vi "Check If Calibration Data Exist.vi"(9 "Set Pressures List":dbl[][](array[numeric])=[[665.1538332158755, 622.4106177021335]], 10 "Mix Cluster":T2, 11 "Calibration Refs":T1) -> (1 "Calibration Data Exists?":bool, 2 "Pressure For Mix 2":dbl[](array[numeric]), 3 "Pressure For Mix 1":dbl[](array[numeric]))   [LabVIEW 2016]
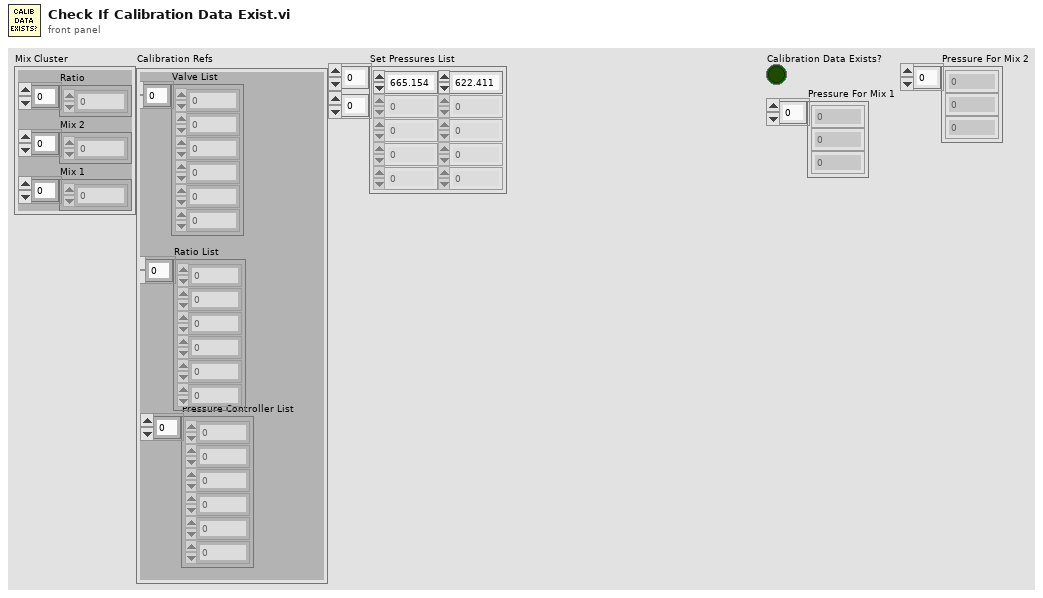
[diagram p1: front panel]
types:
  T1 = cluster{"Pressure Controller List":u8[], "Ratio List":dbl[], "Valve List":u16[]}
  T2 = cluster{"Ratio":dbl[], "Mix 2":u16[], "Mix 1":u16[]}
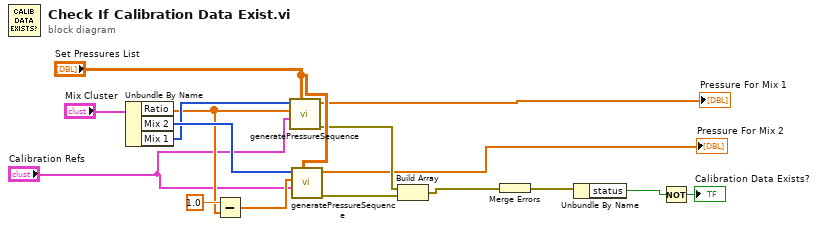
[diagram p0: block diagram]
diagram:
  n1 = Unbundle By Name("Mix Cluster") -> ("Ratio"=w12:dbl[], "Mix 2"=w15:u16[], "Mix 1"=w14:u16[])
  n2 = Subtract(x=1.0, y=w12) -> (x-y=w11:dbl[])
  n3 = call "generatePressureSequence.vi"("Set Pressures List"="Set Pressures List", "Calibration Refs"="Calibration Refs", "Ratio"=w12, "Mix"=w14) -> ("error out"=w7:errorcluster, "Pressure For Mix"=→"Pressure For Mix 1":dbl[])  [unwired: 3 in, 3 out]
  n4 = call "generatePressureSequence.vi"("Set Pressures List"="Set Pressures List", "Calibration Refs"="Calibration Refs", "Ratio"=w11, "Mix"=w15) -> ("error out"=w8:errorcluster, "Pressure For Mix"=→"Pressure For Mix 2":dbl[])  [unwired: 3 in, 3 out]
  n5 = Build Array(w7, w8) -> (w6:errorcluster[])
  n6 = Merge Errors(w6) -> (w5:errorcluster)
  n7 = Unbundle By Name(w5) -> ("status"=w4:bool)
  n8 = Not(x=w4) -> (.not. x?=→"Calibration Data Exists?":bool)
